vi "Is Above or Below Treshold.vi"(8 "error in (no error)":errorcluster, 10 "Keyed Tresholds":refnum<class "1D Array u32.lvclass">, 11 "Line Profiles":refnum<class "2D Array f32.lvclass">) -> (0 "error out":errorcluster, 3 "Is Below Treshold?":refnum<class "2D Array binary.lvclass">)   [LabVIEW 2020, in "G2CPU Line Profile.lvlib"]
uses:
  G2CPU Line Profile.lvlib
  <vilib>/Natan Biesmans/G2CPU GPU and CPU HPC Toolkit/G2CPU Libraries/Arrays/1DArray/u32/1D Array u32.lvclass
  C:/Program Files/National Instruments/LabVIEW 2025/vi.lib/Natan Biesmans/G2CPU GPU and CPU HPC Toolkit/G2CPU Libraries/Arrays/Array/Array Prototype.lvclass
  <vilib>/Natan Biesmans/G2CPU GPU and CPU HPC Toolkit/G2CPU Libraries/Arrays/2DArray/f32/2D Array f32.lvclass
  <vilib>/Natan Biesmans/G2CPU GPU and CPU HPC Toolkit/G2CPU Libraries/Arrays/2DArray/binary/2D Array binary.lvclass
  <vilib>/Natan Biesmans/G2CPU GPU and CPU HPC Toolkit/G2CPU Libraries/Arrays/Array/Array Prototype.lvclass/Array Prototype.ctl
  5776cf5d-939b-4453-8dcd-aac7dfde1cdf.vi
  5fd164f7-6b9a-46b6-bc66-cb6e460ff033.vi
  5ce5b56c-3b20-4a56-bc79-0d5737d67307.vi
  c36678bc-5f03-4585-a837-a0723e1fdfb0.vi
  42383014-10e9-4668-a95b-8687a809a05c.vi
  <vilib>/Natan Biesmans/G2CPU GPU and CPU HPC Toolkit/G2CPU Libraries/Arrays/Array/G2CPU Get Array Pointer.vi
  5776cf5d-939b-4453-8dcd-aac7dfde1cdf.vi/d8e2d9cc-c923-495e-b121-b6b84788c73f.vi
  5776cf5d-939b-4453-8dcd-aac7dfde1cdf.vi/345e91f0-9a5e-4de4-af9c-133346717e4a.vi
  5fd164f7-6b9a-46b6-bc66-cb6e460ff033.vi/e9bebd79-1c27-4fc1-b91f-30516104c7f0.vi
  5ce5b56c-3b20-4a56-bc79-0d5737d67307.vi/1bf6e03b-eb75-45f6-9764-49dc38a3a024.vi
  5ce5b56c-3b20-4a56-bc79-0d5737d67307.vi/2da4419f-02df-47a7-be00-1b7e0871fa33.vi
  c36678bc-5f03-4585-a837-a0723e1fdfb0.vi/e9bebd79-1c27-4fc1-b91f-30516104c7f0.vi
  42383014-10e9-4668-a95b-8687a809a05c.vi/ce577589-e75d-42be-a3c5-f5395febe2a6.vi
  42383014-10e9-4668-a95b-8687a809a05c.vi/d13051aa-bce5-446f-b44f-e7ab7cfb1f03.vi
  42383014-10e9-4668-a95b-8687a809a05c.vi/ca2a5711-2ea0-41ce-865a-169a0e3bc9ca.vi
  5ce5b56c-3b20-4a56-bc79-0d5737d67307.vi/1bf6e03b-eb75-45f6-9764-49dc38a3a024.vi/3e802c67-fb96-46a3-ae13-4994a8508b4f.vi
  5ce5b56c-3b20-4a56-bc79-0d5737d67307.vi/1bf6e03b-eb75-45f6-9764-49dc38a3a024.vi/5a50fc67-79e7-4972-80c2-92243cd53dd4.vi
  5ce5b56c-3b20-4a56-bc79-0d5737d67307.vi/2da4419f-02df-47a7-be00-1b7e0871fa33.vi/730f6c57-5c0b-4ee9-b61e-75067b25222b.vi
  5ce5b56c-3b20-4a56-bc79-0d5737d67307.vi/2da4419f-02df-47a7-be00-1b7e0871fa33.vi/096b8799-7810-404e-baca-ba9279cec4bd.vi
  5ce5b56c-3b20-4a56-bc79-0d5737d67307.vi/2da4419f-02df-47a7-be00-1b7e0871fa33.vi/0f1a5a47-bcc5-4796-ac31-8dfcfbc0d7d1.vi
  5ce5b56c-3b20-4a56-bc79-0d5737d67307.vi/2da4419f-02df-47a7-be00-1b7e0871fa33.vi/89f12e17-3330-4b72-ad8f-8dd636660732.vi
  42383014-10e9-4668-a95b-8687a809a05c.vi/d13051aa-bce5-446f-b44f-e7ab7cfb1f03.vi/e7247370-a01f-465a-ac0e-4dfefcb1bb87.vi
  42383014-10e9-4668-a95b-8687a809a05c.vi/d13051aa-bce5-446f-b44f-e7ab7cfb1f03.vi/345e91f0-9a5e-4de4-af9c-133346717e4a.vi
  <vilib>/Natan Biesmans/G2CPU GPU and CPU HPC Toolkit/ArrayFire Driver/VIs/cast.vi
  <vilib>/Natan Biesmans/G2CPU GPU and CPU HPC Toolkit/G2CPU Libraries/Arrays/Array/G2CPU Set Array Pointer.vi
  <vilib>/Natan Biesmans/G2CPU GPU and CPU HPC Toolkit/G2CPU Libraries/Arrays/Array/G2CPU Release Array.vi
  <vilib>/Natan Biesmans/G2CPU GPU and CPU HPC Toolkit/ArrayFire Driver/VIs/transpose.vi
  <vilib>/Natan Biesmans/G2CPU GPU and CPU HPC Toolkit/G2CPU Libraries/Arrays/SubVI/is 2D.vi
  <vilib>/Natan Biesmans/G2CPU GPU and CPU HPC Toolkit/ArrayFire Driver/VIs/sub.vi
  <vilib>/Natan Biesmans/G2CPU GPU and CPU HPC Toolkit/ArrayFire Driver/VIs/sign.vi
  <vilib>/Natan Biesmans/G2CPU GPU and CPU HPC Toolkit/G2CPU Libraries/Arrays/Array/Array Prototype.lvclass
  <vilib>/Natan Biesmans/G2CPU GPU and CPU HPC Toolkit/G2CPU Libraries/Arrays/DataTypes/f32/f32.lvclass
  <vilib>/Natan Biesmans/G2CPU GPU and CPU HPC Toolkit/G2CPU Libraries/Arrays/2DArray/2D Array Prototype.lvclass
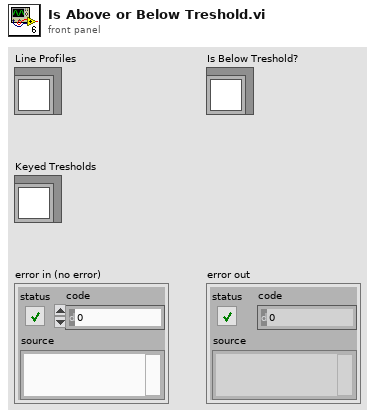
[diagram p1: front panel]
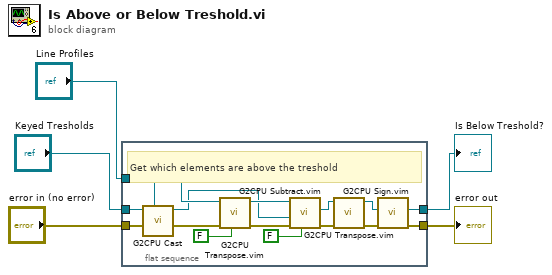
[diagram p0: block diagram]
diagram:
  n1 = flat-sequence {
    tunnel: "Line Profiles" -> [w9]
    tunnel: [w20] -> w5
    tunnel: [w19] -> w1
    tunnel: "error in (no error)" -> [w10]
    tunnel: "Keyed Tresholds" -> [w6]
    frame #0 {
      # "Get which elements are above the treshold"
      n2 = call "G2CPU Cast"("Datatype Prototype"=w9, "error in (no error)"=w10, "Array In"=w6) -> ("error out"=w7:errorcluster, "Array Out"=w8:refnum<class "2D Array f32.lvclass">)  [unwired: 7 in]
      n3 = call "G2CPU Transpose.vim"("Auto Release (Enabled)"=FALSE, "error in (no error)"=w7, "Array In"=w9) -> ("error out"=w15:errorcluster, "Array out"=w14:refnum<class "2D Array f32.lvclass">)  [unwired: 7 in]
      n4 = call "G2CPU Subtract.vim"("Auto Release lhs (Enabled)"=FALSE, "error in (no error)"=w15, "Array rhs"=w8, "Array lhs"=w14) -> ("error out"=w17:errorcluster, "Array Result"=w16:refnum<class "2D Array f32.lvclass">)  [unwired: 6 in]
      n5 = call "G2CPU Transpose.vim"("error in (no error)"=w17, "Array In"=w16) -> ("error out"=w13:errorcluster, "Array out"=w12:refnum<class "2D Array f32.lvclass">)  [unwired: 8 in]
      n6 = call "G2CPU Sign.vim"("error in (no error)"=w13, "Array in"=w12) -> ("error out"=w20:errorcluster, "Array Result"=w19:refnum<class "2D Array binary.lvclass">)  [unwired: 8 in]
    }
  }
  "error out" <- w5
  "Is Below Treshold?" <- w1
